vi "Scale 1D PtByPt.vi"(4 "initialize":bool, 5 "sample length":i32=100, 6 "x":dbl format="%0.2f") -> (0 "error":i32, 1 "offset":dbl format="%0.2f", 2 "scale":dbl format="%0.2f", 3 "Y=(X-offset)/scale":dbl[](array[numeric]))   [LabVIEW 2020, in "NI_PtbyPt.lvlib"]
doc: "Determines <B>scale</B> and <B>offset</B> and scales the set of input data specified by <B>sample length</B> using these values."
uses:
  <vilib>/ptbypt/NI_PtbyPt.lvlib
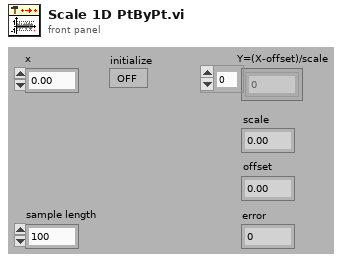
[diagram p1: front panel]
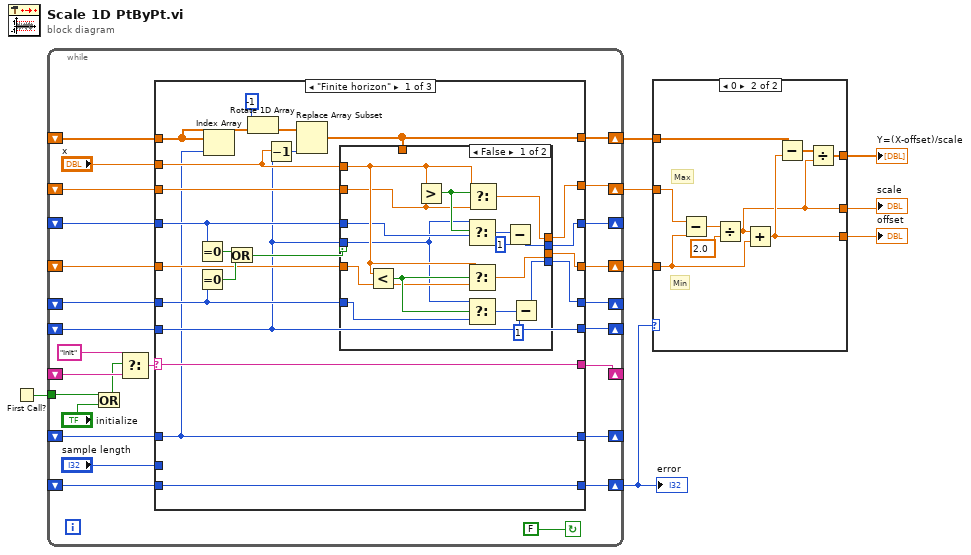
[diagram p0: block diagram]
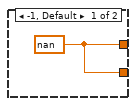
[diagram p2: hidden frame]
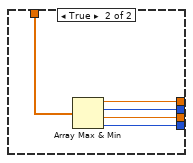
[diagram p3: hidden frame]
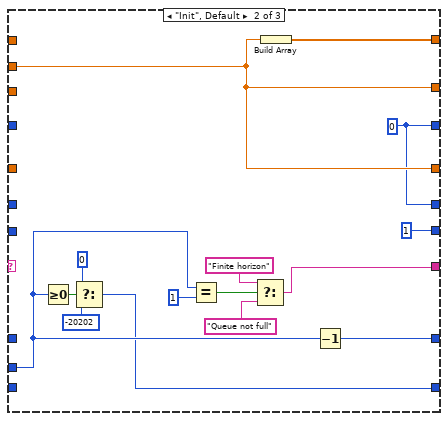
[diagram p4: hidden frame]
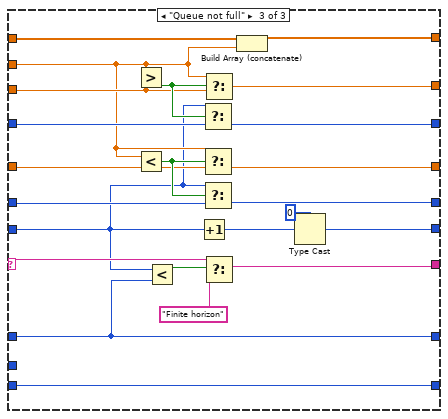
[diagram p5: hidden frame]
diagram:
  n1 = First Call?() -> (First Call?: T/F=w8:bool)
  n2 = while {
    shift-left: _ -> [w11]
    shift-right: [w12] -> _
    tunnel: w8 -> [w15]
    shift-left: _ -> [w19]
    shift-right: [w22] -> w6
    shift-left: _ -> [w20]
    shift-right: [w21] -> _
    shift-left: _ -> [w24]
    shift-right: [w23] -> w7
    shift-left: _ -> [w26]
    shift-right: [w25] -> w5
    shift-left: _ -> [w28]
    shift-right: [w29] -> _
    shift-left: _ -> [w30]
    shift-right: [w31] -> _
    shift-left: _ -> [w34]
    shift-right: [w27] -> _
    shift-right: [w10] -> w1
    shift-left: _ -> [w9]
    stop <- FALSE continue-if-true
    n3 = Or(x=w15, y="initialize") -> (x .or. y?=w13:bool)
    n4 = Select(t="Init", s=w13, f=w34) -> (s? t:f=w32:string)
    n5 = case shown="\"Finite horizon\"" w32 {
      selector: w32 -> [w52 _ w108]
      tunnel: [w38 w85 w99] -> w31
      tunnel: w30 -> [w40 _ w100]
      tunnel: "x" -> [w44 w86 w95]
      tunnel: [w39 1 w111] -> w29
      tunnel: w28 -> [w39 _ w94]
      tunnel: [w52 w79 w106] -> w27
      tunnel: w26 -> [w46 _ w114]
      tunnel: [w45 w78 w113] -> w25
      tunnel: "sample length" -> [_ w81 _]
      tunnel: w24 -> [w43 _ w103]
      tunnel: [w48 w86 w96] -> w23
      tunnel: [w47 w86 w98] -> w22
      tunnel: [w37 w85 w97] -> w21
      tunnel: w20 -> [w42 _ w102]
      tunnel: w19 -> [w41 _ w101]
      tunnel: [w36 w80 w93] -> w12
      tunnel: w11 -> [w36 _ w93]
      tunnel: [w35 w77 w92] -> w10
      tunnel: w9 -> [w35 _ w92]
      frame "Finite horizon" {
        n6 = Equal To 0?(x=w42) -> (x = 0?=w51:bool)
        n7 = Equal To 0?(x=w40) -> (x = 0?=w50:bool)
        n8 = Index Array(array=w46, index=w36) -> ()  [unwired: 1 out]
        n9 = Or(x=w51, y=w50) -> (x .or. y?=w49:bool)
        n10 = Rotate 1D Array(1:w46, 2:i16 -1 ("n")) -> (0:w54:dbl[])
        n11 = Decrement(x=w39) -> (x-1=w53:i32)
        n12 = Replace Array Subset(array=w54, new element=w44, index=w53) -> (w45:dbl[])
        n13 = case shown="False" w49 {
          tunnel: w45 -> [_ w76]
          tunnel: [w64 w75] -> w48
          tunnel: [w60 w74] -> w37
          tunnel: [w63 w73] -> w47
          tunnel: [w56 w72] -> w38
          tunnel: w44 -> [w69 _]
          tunnel: w43 -> [w68 _]
          tunnel: w42 -> [w65 _]
          tunnel: w41 -> [w67 _]
          tunnel: w40 -> [w66 _]
          tunnel: w39 -> [w62 _]
          frame False {
            n14 = Less?(x=w69, y=w67) -> (x < y?=w70:bool)
            n15 = Greater?(x=w69, y=w68) -> (0:w71:bool)
            n16 = Select(t=w62, s=w71, f=w65) -> (s? t:f=w61:i32)
            n17 = Select(t=w69, s=w70, f=w67) -> (s? t:f=w63:dbl)
            n18 = Select(t=w62, s=w70, f=w66) -> (s? t:f=w58:i32)
            n19 = Select(t=w69, s=w71, f=w68) -> (s? t:f=w64:dbl)
            n20 = Subtract(x=w61, y=1) -> (x-y=w60:i32)
            n21 = Subtract(x=w58, y=1) -> (x-y=w56:i32)
          }
          frame True {
            n22 = Array Max & Min(array=w76) -> (max value=w75:dbl, max index (indices)=w74:i32, min value=w73:dbl, min index (indices)=w72:i32)
          }
        }
      }
      frame "Init", Default {
        w85 = 0
        n23 = Greater Or Equal To 0?(x=w81) -> (x >= 0?=w84:bool)
        n24 = Select(t=0, s=w84, f=-20202) -> (s? t:f=w77:i32)
        n25 = Equal?(x=w81, y=1) -> (x = y?=w89:bool)
        n26 = Select(t="Finite horizon", s=w89, f="Queue not full") -> (s? t:f=w79:string)
        n27 = Build Array(w86) -> (w78:dbl[])
        n28 = Decrement(x=w81) -> (x-1=w80:i32)
      }
      frame "Queue not full" {
        n29 = Greater?(x=w95, y=w103) -> (0:w105:bool)
        n30 = Less?(x=w95, y=w101) -> (x < y?=w104:bool)
        n31 = Less?(x=w94, y=w93) -> (x < y?=w109:bool)
        n32 = Increment(x=w94) -> (x+1=w112:i32)
        n33 = Select(t=w94, s=w105, f=w102) -> (s? t:f=w97:i32)
        n34 = Select(t=w95, s=w104, f=w101) -> (s? t:f=w98:dbl)
        n35 = Select(t=w94, s=w104, f=w100) -> (s? t:f=w99:i32)
        n36 = Select(t=w95, s=w105, f=w103) -> (s? t:f=w96:dbl)
        n37 = Select(t=w108, s=w109, f="Finite horizon") -> (s? t:f=w106:string)
        n38 = Build Array (concatenate)(w114, w95) -> (w113:dbl[])
        n39 = Type Cast(type=0, x=w112) -> (*(type *) &x=w111:i32)
      }
    }
  }
  "error" <- w1
  n40 = case shown="0" w1 {
    tunnel: w7 -> [_ w122]
    tunnel: w6 -> [_ w121]
    tunnel: w5 -> [_ w120]
    tunnel: [w115 w119] -> w4
    tunnel: [w115 w117] -> w3
    tunnel: [_ w116] -> w2
    frame -1, Default {
      w115 = nan
    }
    frame 0 {
      # "Min"
      # "Max"
      n41 = Subtract(x=w122, y=w121) -> (x-y=w124:dbl)
      n42 = Divide(x=w124, y=2.0) -> (x/y=w117:dbl)
      n43 = Add(x=w117, y=w121) -> (x+y=w119:dbl)
      n44 = Subtract(x=w120, y=w119) -> (x-y=w118:dbl[])
      n45 = Divide(x=w118, y=w117) -> (x/y=w116:dbl[])
    }
  }
  "Y=(X-offset)/scale" <- w2
  "scale" <- w3
  "offset" <- w4
